vi "Write CAN Frames.vi"(7 "Channel Number":u32, 8 "error in (no error)":errorcluster, 9 "Timeout (ms)":i32=100, 10 "Frames":T1[](array[typedef]) {"payload" format="%x"; "timestamp" format="%<%.7X\n%x>T"; "type" items=["CAN Data"=0, "CAN Remote"=1, "CAN Bus Error"=2, "CAN 2.0 Data"=8, "CAN FD Data"=16, "CAN FD+BRS Data"=24, "J1939 Data"=192, "Delay"=224, "Log Trigger"=225, "Start Trigger"=226]; "identifier" format="%x"}, 11 "FPGA Refnum":T3) -> (0 "error out":errorcluster)   [LabVIEW 2020, in "985x Support Addon Engine.lvlib"]
uses:
  985x Support Addon Engine.lvlib
  Types/FPGA Refnum.ctl
  <vilib>/xnet/xnet.llb/XNET Frame CAN.ctl
  <vilib>/xnet/xnet.llb/XNET Frame Type CAN.ctl
  <vilib>/Utility/error.llb/Error Cluster From Error Code.vi
  <vilib>/rvi/errors/niLvFpgaAdjustHostInterfaceError.vi
  <vilib>/rvi/interface/nirviMethod/nirviMethod.xnode
  <vilib>/FPGAPlugInAG/Dynamic/niLvFpga_WriteFifo_Dynamic.vi
  <vilib>/rvi/errors/niLvFpgaMergeErrorWithErrorCode.vi
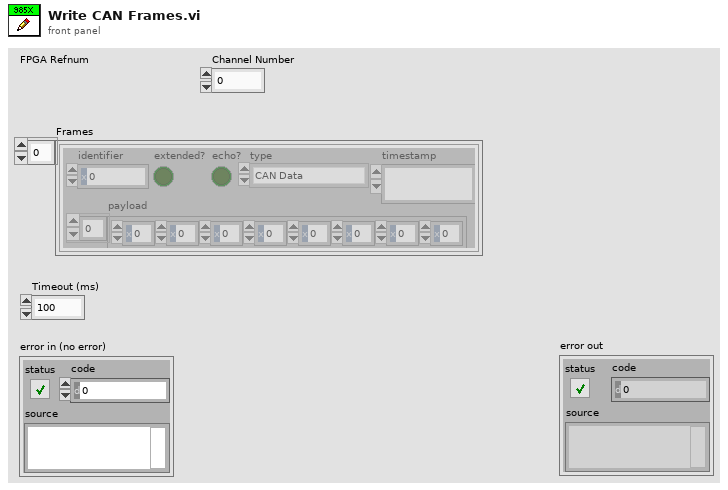
[diagram p1: front panel]
types:
  T1 = typedef "XNET Frame CAN.ctl" = cluster{"timestamp":timestamp, "payload":u8[], "identifier":u32, "type":T2, "extended?":bool, "echo?":bool}
  T2 = typedef "XNET Frame Type CAN.ctl" = u8
  T3 = typedef "985x Support Addon Engine.lvlib/FPGA Refnum.ctl" = refnum<k20>
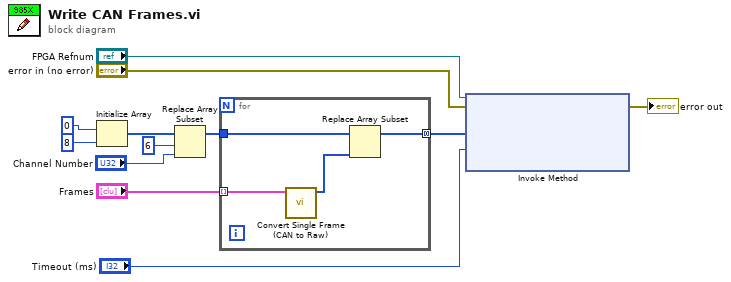
[diagram p0: block diagram]
diagram:
  n1 = Initialize Array(u32 0, 8 ("dimension size")) -> (w8:u32[])
  n2 = Replace Array Subset(array=w8, new element="Channel Number", index=6) -> (w6:u32[])
  n3 = for {
    tunnel: "Frames" -> [w16] mode=indexing
    tunnel: w6 -> [w15]
    tunnel: [w13] -> w4 mode=concatenating
    n4 = call "Convert Single Frame (CAN to Raw).vi"("CAN frame"=w16) -> ("Raw U32"=w14:u32[])  [unwired: 9 in, 1 out]
    n5 = Replace Array Subset(array=w15, new element=w14) -> (w13:u32[])  [unwired: 1 in]
  }
  n6 = xnode "Invoke Method"("FPGA VI Reference In"="FPGA Refnum", "error in"="error in (no error)", "Data"=w4, "Timeout (ms)"="Timeout (ms)") -> ("error out"=→"error out":errorcluster)  [unwired: 2 out]
